vi "destroy.vi"(0 "vector_qdrant in":refnum<class "vector_qdrant.lvclass">, 11 "error in (no error)":errorcluster) -> (4 "vector_qdrant out":refnum<class "vector_qdrant.lvclass">, 15 "error out":errorcluster)   [LabVIEW 2020, in "vector_qdrant.lvclass"]
uses:
  vector_qdrant.lvclass
  vector_qdrant.lvclass/vector_qdrant.ctl
  abstract_vector_base/abstract_vector_base.lvclass
  <vilib>/httpClient/LabVIEWHTTPClient.lvlib
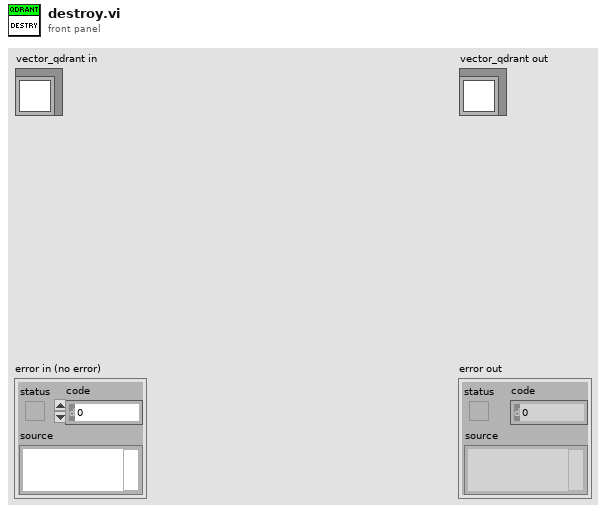
[diagram p1: front panel]
types:
  T1 = typedef "LabVIEWHTTPClient.lvlib/ClientHandle.ctl" = refnum<k1>
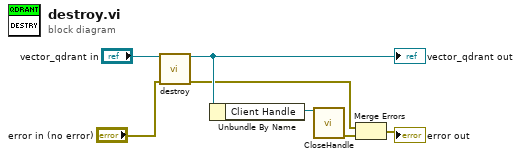
[diagram p0: block diagram]
diagram:
  n1 = call-parent "destroy.vi"("abstract_vector_base in"="vector_qdrant in", "error in (no error)"="error in (no error)") -> ("abstract_vector_base out"=w5:refnum<class "vector_qdrant.lvclass">, "error out"=w1:errorcluster)  [unwired: 12 in]
  "vector_qdrant out" <- w5
  n2 = Unbundle By Name(w5) -> ("Client Handle"=w4:T1)
  n3 = call <vilib>:"CloseHandle.vi"("client handle"=w4) -> ("error out"=w3:errorcluster)  [unwired: 14 in]
  n4 = Merge Errors(w1, w3) -> (→"error out":errorcluster)
